vi "Frame Error.vi"(0 "Error List":string[](array[string]), 11 "Error In":errorcluster) -> (4 "Error Code":i32=5001, 6 "Error Message":string, 15 "Error Out":errorcluster)   [LabVIEW 2024, in "devicePowerSequencerCoreLogic.lvlib"]
doc: "Builds the custom error based on the input error string and Error In input"
uses:
  devicePowerSequencerCoreLogic.lvlib
  <vilib>/Utility/error.llb/DialogType.ctl
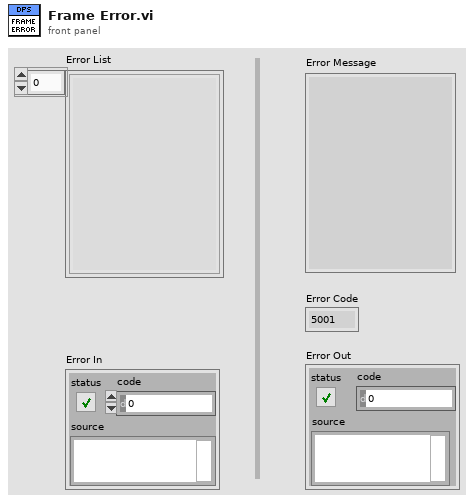
[diagram p1: front panel]
types:
  T1 = typedef "DialogType.ctl" = u16
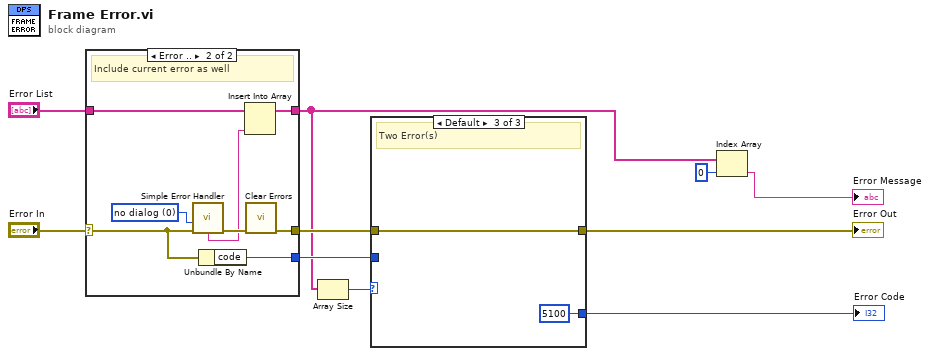
[diagram p0: block diagram]
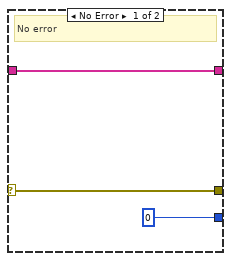
[diagram p2: hidden frame]
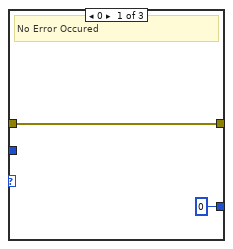
[diagram p3: hidden frame]
diagram:
  n1 = case shown="Error .." "Error In" {
    selector: "Error In" -> [w13 w15]
    tunnel: [w13 w19] -> w8
    tunnel: "Error List" -> [w12 w18]
    tunnel: [w12 w17] -> w4
    tunnel: [0 ("code") w14] -> w5
    frame No Error {
      # "No error"
    }
    frame Error {
      w21 = T1 0 items=["no dialog", "OK message", "continue or stop message", "OK message + warnings", "continue/stop + warnings"] ("type of dialog (OK msg:1)")
      # "Include current error as well"
      n2 = call <vilib>:"Simple Error Handler.vi"("type of dialog (OK msg:1)"=w21, "error in (no error)"=w15) -> ("error out"=w20:errorcluster, "message"=w16:string)  [unwired: 3 in, 3 out]
      n3 = Unbundle By Name(w15) -> ("code"=w14:i32)
      n4 = Insert Into Array(array=w18, new element=w16) -> (w17:string[])  [unwired: 1 in]
      n5 = call <vilib>:"Clear Errors.vi"("error in (no error)"=w20) -> ("error out"=w19:errorcluster)  [unwired: 5 in, 1 out]
    }
  }
  n6 = Array Size(array=w4) -> (size(s)=w10:i32)
  n7 = case shown="Default" w10 {
    tunnel: w8 -> [w23 w24 w26]
    tunnel: [w23 w24 w26] -> w1
    tunnel: [0 ("Error Code") _ 5100 ("code")] -> w6
    tunnel: w5 -> [_ _ _]
    frame 0 {
      # "No Error Occured"
    }
    frame 1 {
    }
    frame Default {
      # "Two Error(s)"
    }
  }
  "Error Out" <- w1
  "Error Code" <- w6
  n8 = Index Array(array=w4, index=0) -> (element=→"Error Message":string)
